vi "Invalid Response.vi"(5 "error source class name":string, 7 "error source vi name":string, 8 "error in (no error)":errorcluster, 9 "actual response":string, 10 "expected response":string, 11 "Interface in":refnum<class "Interface.lvclass">) -> (0 "error out":errorcluster, 3 "Interface out":refnum<class "Interface.lvclass">)   [LabVIEW 2017, in "DSF Core.lvlib" / "Interface.lvclass"]
uses:
  Interface/Interface.lvclass
  Interface/Errors.ctl
  <vilib>/NI/Memory Manager/Static Error Handling.lvlib
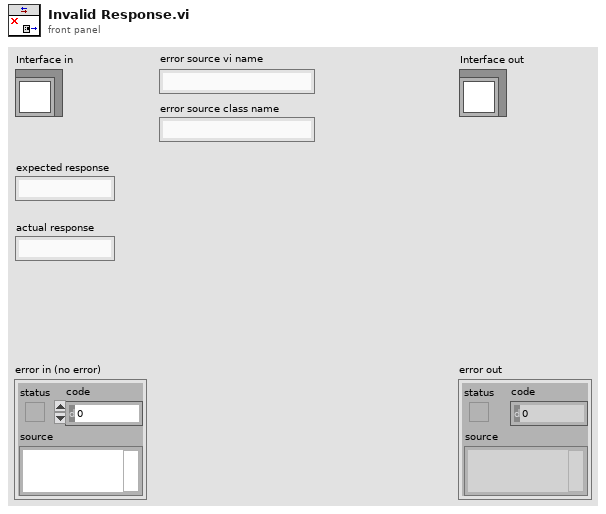
[diagram p1: front panel]
types:
  T1 = typedef "DSF Core.lvlib/Interface.lvclass/Errors.ctl" = enum16{"Command Timeout", "Response Timeout", "Error Timeout", "Invalid Response", "Invalid Response Parameters"}
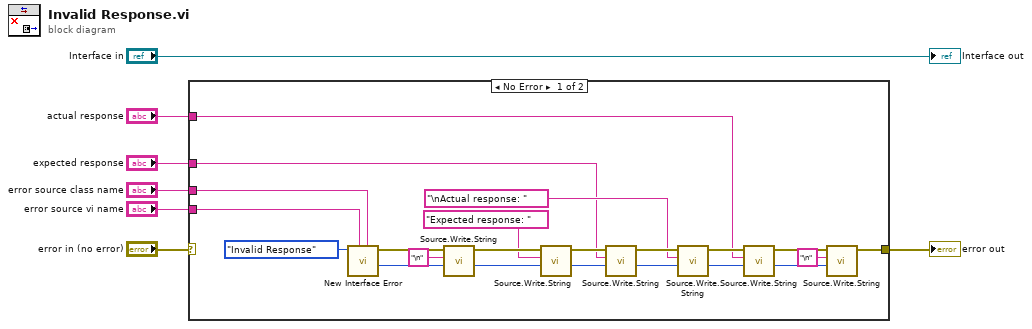
[diagram p0: block diagram]
diagram:
  n1 = case shown="No Error" "error in (no error)" {
    selector: "error in (no error)" -> [_ w30]
    tunnel: [w12 w30] -> w5
    tunnel: "error source vi name" -> [w29 _]
    tunnel: "actual response" -> [w11 _]
    tunnel: "expected response" -> [w10 _]
    tunnel: "error source class name" -> [w8 _]
    frame No Error {
      n2 = call "New Interface Error.vi"("error source class name"=w8, "error source vi name"=w29, "error"=Errors."Invalid Response") -> ("new offset"=w27:i32, "error out"=w28:errorcluster)  [unwired: 7 in]
      n3 = call <vilib>:"Source.Write.String.vi"("offset"=w27, "string"="\n", "error in"=w28) -> ("new offset"=w24:i32, "error out"=w25:errorcluster)  [unwired: 7 in]
      n4 = call <vilib>:"Source.Write.String.vi"("offset"=w24, "string"="Expected response: ", "error in"=w25) -> ("new offset"=w23:i32, "error out"=w22:errorcluster)  [unwired: 7 in]
      n5 = call <vilib>:"Source.Write.String.vi"("offset"=w23, "string"=w10, "error in"=w22) -> ("new offset"=w19:i32, "error out"=w20:errorcluster)  [unwired: 7 in]
      n6 = call <vilib>:"Source.Write.String.vi"("offset"=w19, "string"="\nActual response: ", "error in"=w20) -> ("new offset"=w16:i32, "error out"=w17:errorcluster)  [unwired: 7 in]
      n7 = call <vilib>:"Source.Write.String.vi"("offset"=w16, "string"=w11, "error in"=w17) -> ("new offset"=w14:i32, "error out"=w15:errorcluster)  [unwired: 7 in]
      n8 = call <vilib>:"Source.Write.String.vi"("offset"=w14, "string"="\n", "error in"=w15) -> ("error out"=w12:errorcluster)  [unwired: 7 in, 1 out]
    }
    frame Error {
    }
  }
  "error out" <- w5
  "Interface out" <- "Interface in"
